vi "CH_LM Utility SCPI.vi"(0 "Meter Index":i32, 1 "SCPI Command/Query":string, 3 "NofStrings (-1:all)":i32=-1, 5 "error in (no error)":errorcluster, 7 "Timeout / ms (3000)":i32=3000, 9 "Lock Timeout / ms (1000)":i32=1000) -> (11 "Lock timed out":bool, 14 "Meter Index":i32, 15 "Response":string, 17 "Response Array":string[](array[string]), 19 "error out":errorcluster)   [LabVIEW 2017, in "CH_LM.lvlib"]
doc: "This VI will send SCPI commands and display messages received for SCPI queries."
uses:
  CH_LM.lvlib
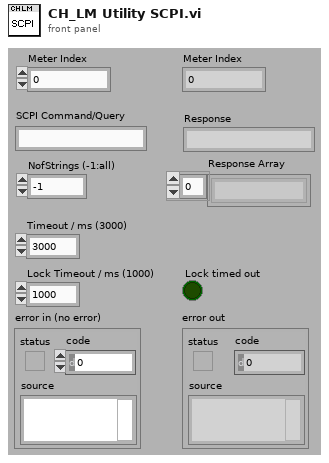
[diagram p1: front panel]
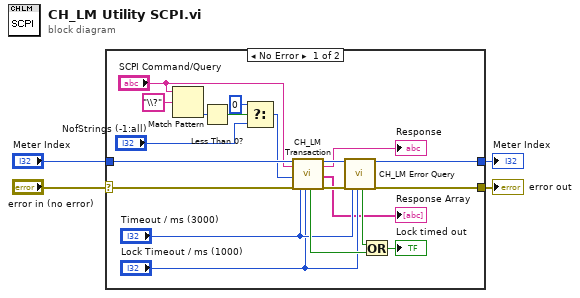
[diagram p0: block diagram]
diagram:
  n1 = case shown="No Error" "error in (no error)" {
    selector: "error in (no error)" -> [w24 w26]
    tunnel: [w19 w26] -> w4
    tunnel: "Meter Index" -> [w23 w25]
    tunnel: [w20 w25] -> w1
    frame No Error {
      n2 = Match Pattern(string="SCPI Command/Query", regular expression="\\?") -> (offset past match=w9:i32)  [unwired: 4 out]
      n3 = Less Than 0?(x=w9) -> (x < 0?=w8:bool)
      n4 = Select(t=0, s=w8, f="NofStrings (-1:all)") -> (s? t:f=w5:i32)
      n5 = call "CH_LM Transaction.vi"("Meter Index"=w23, "Command String"="SCPI Command/Query", "NofStrings (-1:all)"=w5, "error in (no error)"=w24, "Timeout / ms (3000)"="Timeout / ms (3000)", "Lock Timeout / ms (1000)"="Lock Timeout / ms (1000)") -> ("Lock timed out"=w17:bool, "Meter Index"=w22:i32, "Response"=→"Response":string, "Response Array"=→"Response Array":string[], "error out"=w21:errorcluster)  [unwired: 9 out]
      n6 = call "CH_LM Error Query.vi"("Meter Index"=w22, "error in (no error)"=w21, "Timeout / ms (3000)"="Timeout / ms (3000)", "Lock Timeout / ms (1000)"="Lock Timeout / ms (1000)") -> ("Lock timed out"=w18:bool, "Meter Index"=w20:i32, "error out"=w19:errorcluster)  [unwired: 13 out]
      n7 = Or(x=w18, y=w17) -> (x .or. y?=→"Lock timed out":bool)
    }
    frame Error {
    }
  }
  "error out" <- w4
  "Meter Index" <- w1
